vi "State Variable Feedback System.vi"() -> ()   [LabVIEW 2012]
uses:
  <vilib>/Simulation/Scripting/Companion Diagram/SimConfigNode/SimParams.ctl
  <vilib>/Simulation/Scripting/Companion Diagram/SimConfigNode/_simSolvers.ctl
  <vilib>/Simulation/Implementation/Shared/SIMSCR Execution Mode.ctl
  <vilib>/Simulation/Param Hierarchy/Typedefs/SIMPH Param Control Actions.ctl
  <vilib>/Simulation/Implementation/Shared/NILVSim_ParamChanged.vi
  <vilib>/Simulation/ContinuousLinear/Implementation/NILVSim State Space.llb/SIM State Space Distributor (CD).vi
  <vilib>/Simulation/DiscreteLinear/Implementation/NILVSim Discrete Delay.llb/NILVSim Discrete Delay Buffered Distributor (scalar).vi
  <vilib>/Simulation/DiscreteLinear/Implementation/NILVSim Discrete Delay.llb/NILVSim Discrete Delay Buffered Collector (scalar).vi
  <vilib>/Simulation/Implementation/Shared/SIM Is Init or Final Stage.vi
  <vilib>/Simulation/DiscreteLinear/Implementation/NILVSim Discrete Transfer Function Direct.llb/SIM Discrete Transfer Function Direct (SISO).vi
  <vilib>/Simulation/DiscreteLinear/Implementation/NILVSim Discrete Transfer Function Buffered.llb/SIM Discrete Transfer Function Distributor (SISO).vi
  <vilib>/Simulation/ContinuousLinear/Implementation/NILVSim Transfer Function.llb/SIM Transfer Function Collector (SISO).vi
  <vilib>/Simulation/SignalDisplay/Implementation/NILVSim Time Waveform.llb/SIM Time Waveform (vector).vi
  <vilib>/Simulation/ContinuousLinear/Implementation/NILVSim State Space.llb/SIM State Space Collector (CD).vi
  <vilib>/Simulation/Implementation/Shared/NILVSim_Manager.vi
  <vilib>/Simulation/Implementation/Shared/NILVSim_FinalizeModel.vi
  <vilib>/addons/Control Design/_Model Construction/Model Creation.llb/Model Creation SubVI/cd_Create State Space Model.vi
  <vilib>/addons/Control Design/_Time Response Analysis/Time Response.llb/Time Response subVI/cd_Step Response (State-Space).vi
  <vilib>/addons/Control Design/_Dynamic Analysis/Dynamic Analysis.llb/Dynamic Analysis subVI/cd_Poles (State-Space).vi
  <vilib>/Simulation/Implementation/Shared/SIM Unbundle Sim Info.vi
  <vilib>/Utility/error.llb/Clear Errors.vi
  <vilib>/Simulation/Implementation/Shared/NILVSim_GetModelError.vi
  <vilib>/Simulation/Implementation/Shared/SIM Bundle Sim Info.vi
  <vilib>/Simulation/Implementation/Shared/SIMSH Read Queue.vi
  <vilib>/Simulation/Implementation/Shared/NILVSim_Initialize.vi
  <vilib>/addons/Control Design/_Implementation/CD State Feedback Controller.vi
  <vilib>/addons/Control Design/_Implementation/CD State Feedback Controller (Single Output).vi
  <vilib>/Simulation/Utility/Implementation/NILVSim Get Time and IsAcceptedStep.vi
  <vilib>/Simulation/Scripting/Companion Diagram/SimConfigNode/SimDog.xnode
  <vilib>/Simulation/Implementation/XNodeFramework/SimXNode/SimX.xnode
  <vilib>/addons/Control Design/_Model Construction/NI_LinSys_Model Creation.lvlib
  <vilib>/addons/Control Design/_Dynamic Analysis/NI_CD_Dynamic Analysis.lvlib
  <vilib>/addons/Control Design/_Time Response Analysis/NI_CD_Time Response.lvlib
  <vilib>/addons/Control Design/_State Feedback Control/NI_CD_State Feedback Control.lvlib
  <vilib>/Simulation/DiscreteLinear/Implementation/NILVSim Discrete Transfer Function Buffered.llb/SIM Discrete Transfer Function Buffered (SISO).vi
  <vilib>/Simulation/DiscreteLinear/Implementation/NILVSim Discrete Delay.llb/SIM Discrete Delay Buffered (scalar).vi
  <vilib>/addons/Control Design/_Implementation/NI_CD_Implementation.lvlib
  <vilib>/addons/Control Design/_Model Construction/Model Typedefs.llb/CD General Elements.ctl
  <vilib>/addons/Control Design/_Model Construction/NI_LinSys_Model Typedefs.lvlib
  <vilib>/addons/Control Design/_Model Construction/Model Typedefs.llb/CD State Space Model (MIMO).ctl
  <vilib>/Simulation/ContinuousLinear/Implementation/NILVSim State Space.llb/SIM State Space (CD).vi
  <vilib>/Simulation/Implementation/Shared/NI_SIM_Implementation.lvlib
panel:
  out "Outputs":dbl[](array[numeric])
  out "Plot X and Theta":waveform(dbl)[](graph)=[{"t0"=timestamp(4.71 s since 1904-01-01), "dt"=1.0, "Y"=[-0.13996665083491025]}, {"t0"=timestamp(4.71 s since 1904-01-01), "dt"=1.0, "Y"=[-1.62298383744272e-05]}]
  in  "Initial Conditions":T1
  in  "Set Point (m)":dbl(slide)=-0.14 scale=-0.2..0.2
  out "Actual Poles":cdb[](array[numeric]) format="%.2f"
  in  "Gain Type":u16(ring) items=["Controller Gain", "Observer Gain (Predictive)", "Observer Gain (Current)"]
  in  "Desired System Poles":cdb[](array[numeric])=[-5.0+0.0i, -5.0+0.0i, -20.0+0.0i, -15.0+0.0i] format="%.2f"
  out "State Trajectory Graph":cluster{"time":dbl[], dbl[]}[](graph)
  out "Step Response Graph":cluster{"time":dbl[], dbl[]}[](graph)
  out "System Poles":cdb[](array[numeric]) format="%.3f"
  in  "Sampling Time (s)":dbl format="%#.6p"
  in  "D":dbl[][](array[numeric])=[[0.0], [0.0]]
  in  "C":dbl[][](array[numeric])=[[1.0, 0.0, 0.0], [0.0, 0.0, 1.0]]
  in  "H":dbl[][](array[numeric])=[[0.0], [1.82], [0.0], [4.55]]
  in  "G":dbl[][](array[numeric])=[[0.0, 1.0, 0.0, 0.0], [0.0, -0.18, 2.67, 0.0], [0.0, 0.0, 0.0, 1.0], [0.0, -0.45, 31.18, 0.0]]
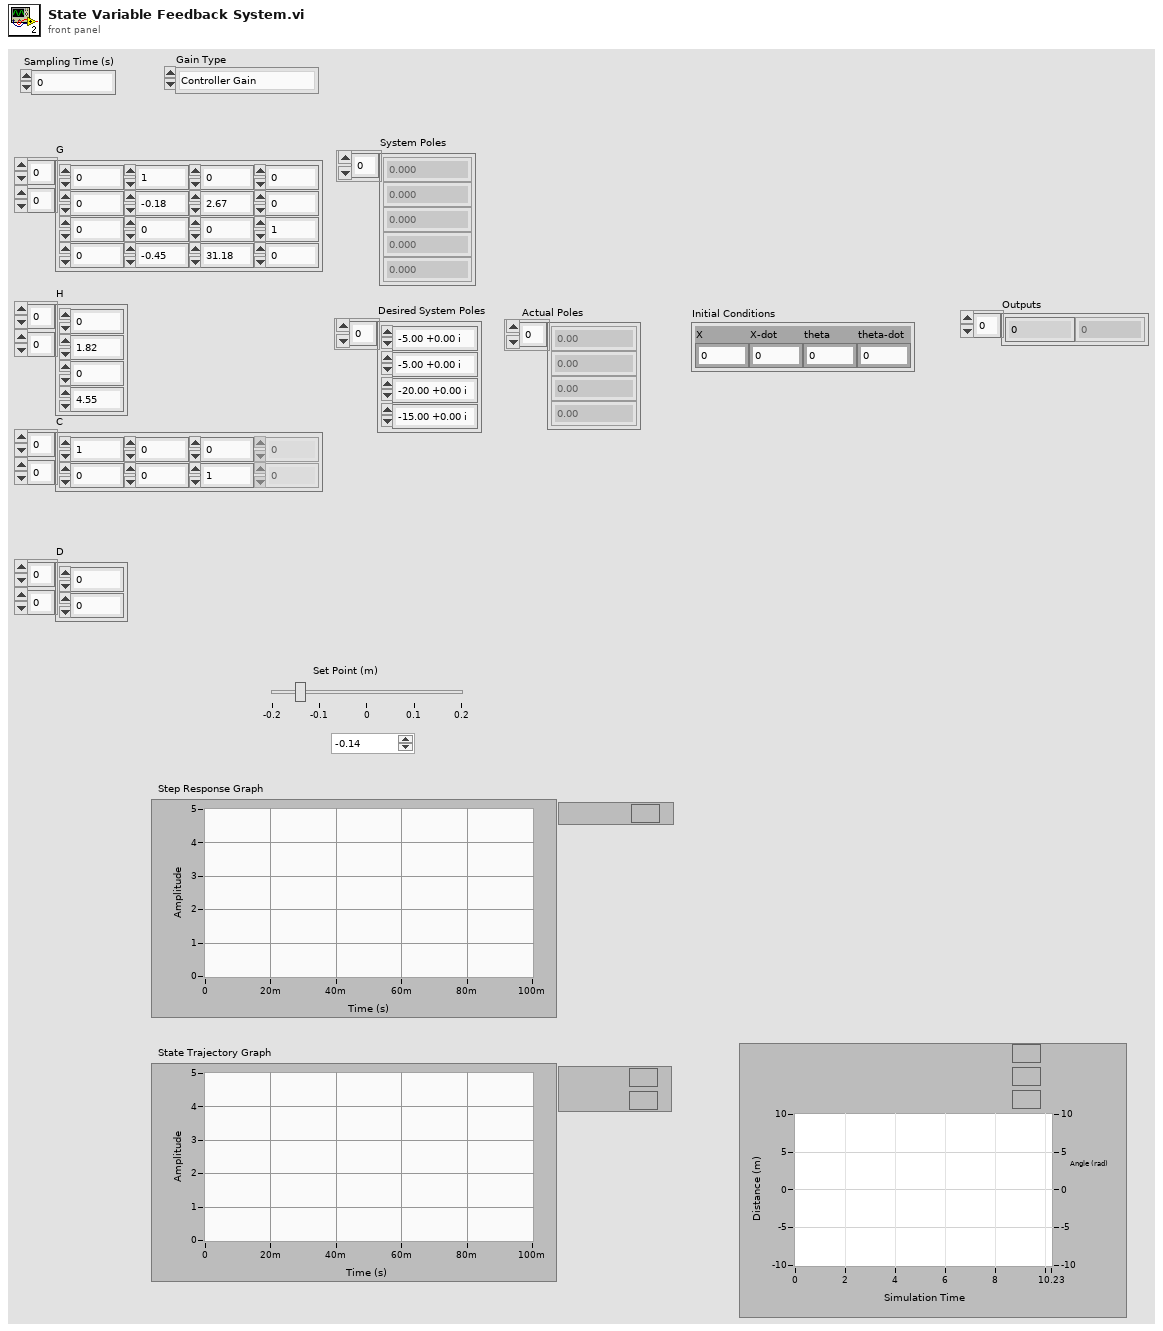
[diagram p1: front panel]
types:
  T1 = cluster{"X":dbl, "X-dot":dbl, "theta":dbl, "theta-dot":dbl}
  T2 = typedef "NI_LinSys_Model Typedefs.lvlib/CD State Space Model (MIMO).ctl" = cluster{"properties":T3, "A":dbl[][], "B":dbl[][], "C":dbl[][], "D":dbl[][], "StateNames":string[], "Transport Delay":dbl[][]}
  T3 = typedef "NI_LinSys_Model Typedefs.lvlib/CD General Elements.ctl" = cluster{"Model name":string, "Input names":string[], "Output names":string[], "Input Delays":dbl[], "Output Delays":dbl[], "Sampling Time":dbl, "Notes":string}
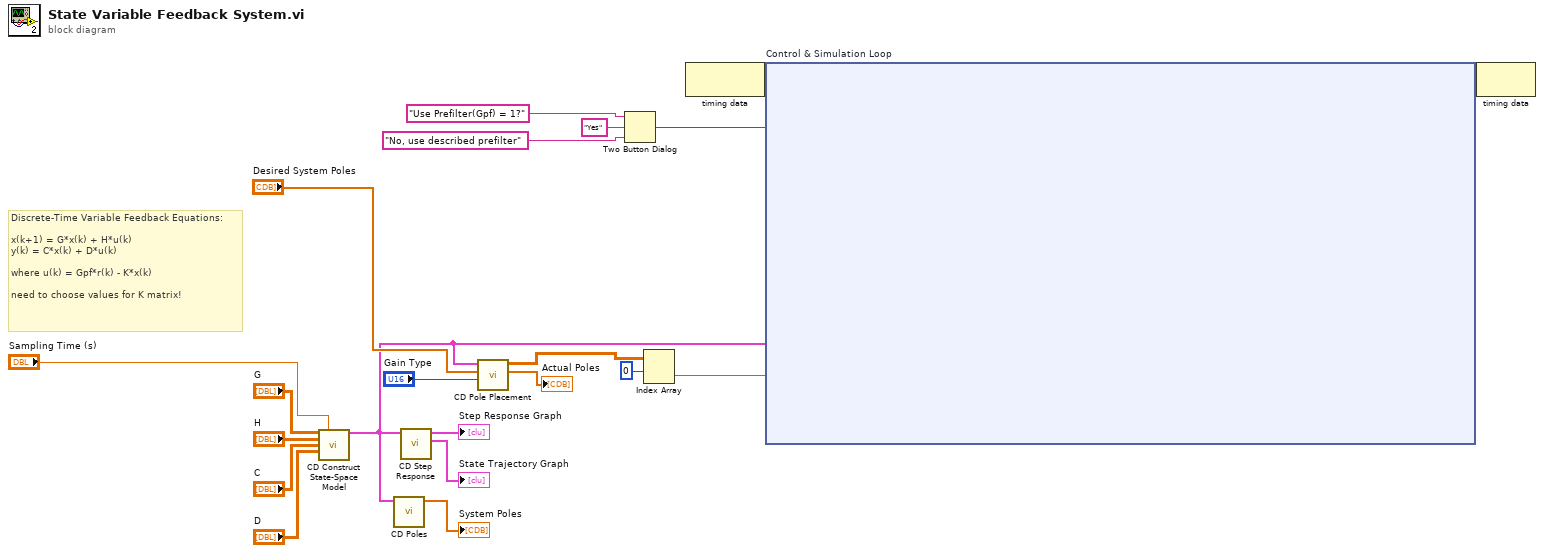
[diagram p0: block diagram]
diagram:
  # "Discrete-Time Variable Feedback Equations:\n\nx(k+1) = G*x(k) + H*u(k)\ny(k) = C*x(k) + D*u(k)\n\nwhere u(k) = Gpf*r(k) - K*x(k)\n\nneed to choose values for K matrix!"
  n1 = call-poly <vilib>:"CD Construct State-Space Model.vi"("A"="G", "Sampling Time (s)"="Sampling Time (s)", "B"="H", "C"="C", "D"="D") -> ("State-Space Model"=w6:T2)  [unwired: 9 in, 1 out]
  n2 = call-poly <vilib>:"CD Poles.vi"("State-Space Model"=w6) -> ("Poles"=→"System Poles":cdb[])  [unwired: 9 in, 1 out]
  n3 = call-poly <vilib>:"CD Step Response.vi"("State-Space Model"=w6) -> ("State Trajectory Graph"=→"State Trajectory Graph":cluster{"time":dbl[], dbl[]}[], "Step Response Graph"=→"Step Response Graph":cluster{"time":dbl[], dbl[]}[])  [unwired: 7 in, 2 out]
  n4 = call <vilib>:"CD Pole Placement.vi"("Gain Type"="Gain Type", "Poles"="Desired System Poles", "State-Space Model"=w6) -> ("Actual Poles"=→"Actual Poles":cdb[], "Gain"=w8:dbl[][])  [unwired: 6 in, 1 out]
  n5 = Two Button Dialog(message="Use Prefilter(Gpf) = 1?", 1:"No, use described prefilter" ("F button name (\"Cancel\")"), 2:"Yes" ("T button name (\"OK\")")) -> (T button?=w2:bool)
  n6 = Index Array(array=w8, index (row)=0) -> (element=w1:dbl[])  [unwired: 1 in]
  n7 = node-c288() -> (w21:variant)  [unwired: 1 in]
  n8 = node-c254 "Control & Simulation Loop"(w21, w1, w6, w2) -> (w20:variant)
  n9 = node-c288(w20) -> ()  [unwired: 1 out]
